vi "Save Waveform To File.vi"(8 "error in":errorcluster, 10 "Waveforms":waveform(dbl)[](array[waveform]), 11 "Measurement Configuration In":T1={"TDMS File Location"="", "Run Action"="Create/Replace Wfm Group", "Wfm Group Name"="Wfm1", "Channel Names"=[], "Waveforms Summary JSON"=[]}) -> (0 "error out":errorcluster, 2 "Final Wfm Group Name":string, 3 "Measurement Configuration Out":T1)   [LabVIEW 2025, in "TDMS Waveform Creator.lvclass"]
uses:
  TDMS Waveform Creator.lvclass
  TDMS Waveform Creator.lvclass/TDMS Waveform Creator.ctl
  <vilib>/regexp/Match Regular Expression.xnode
  <vilib>/ErrorRing/Error Ring.xnode
  <vilib>/Utility/error.llb/Error Cluster From Error Code.vi
  Measurement Configuration.ctl
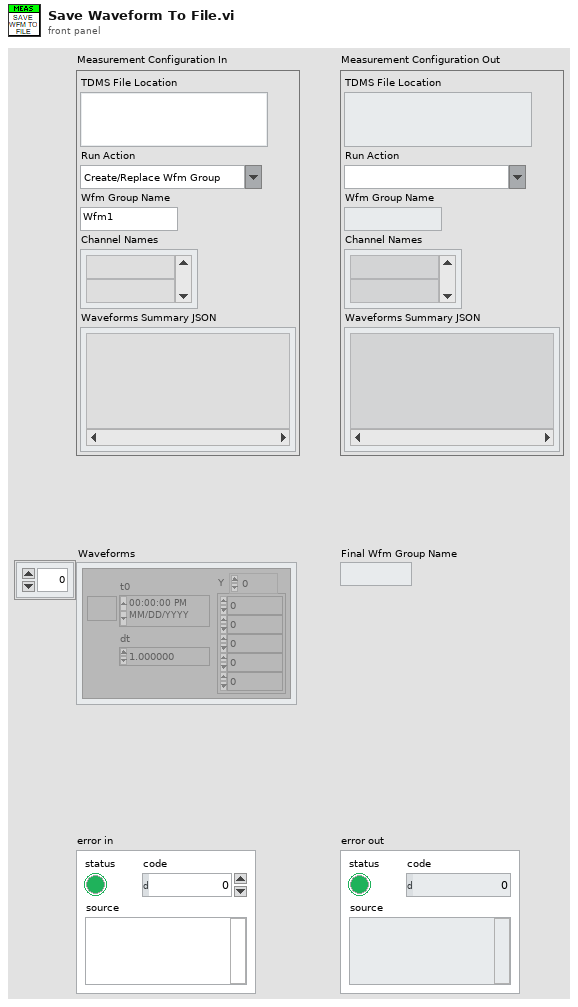
[diagram p1: front panel]
types:
  T1 = typedef "TDMS Waveform Creator.lvclass/Measurement Configuration.ctl" = cluster{"TDMS File Location":string, "Run Action":string, "Wfm Group Name":string, "Channel Names":string[], "Waveforms Summary JSON":string[]}
  T2 = enum16{"open", "open or create", "create or replace", "create", "open (read-only)"}
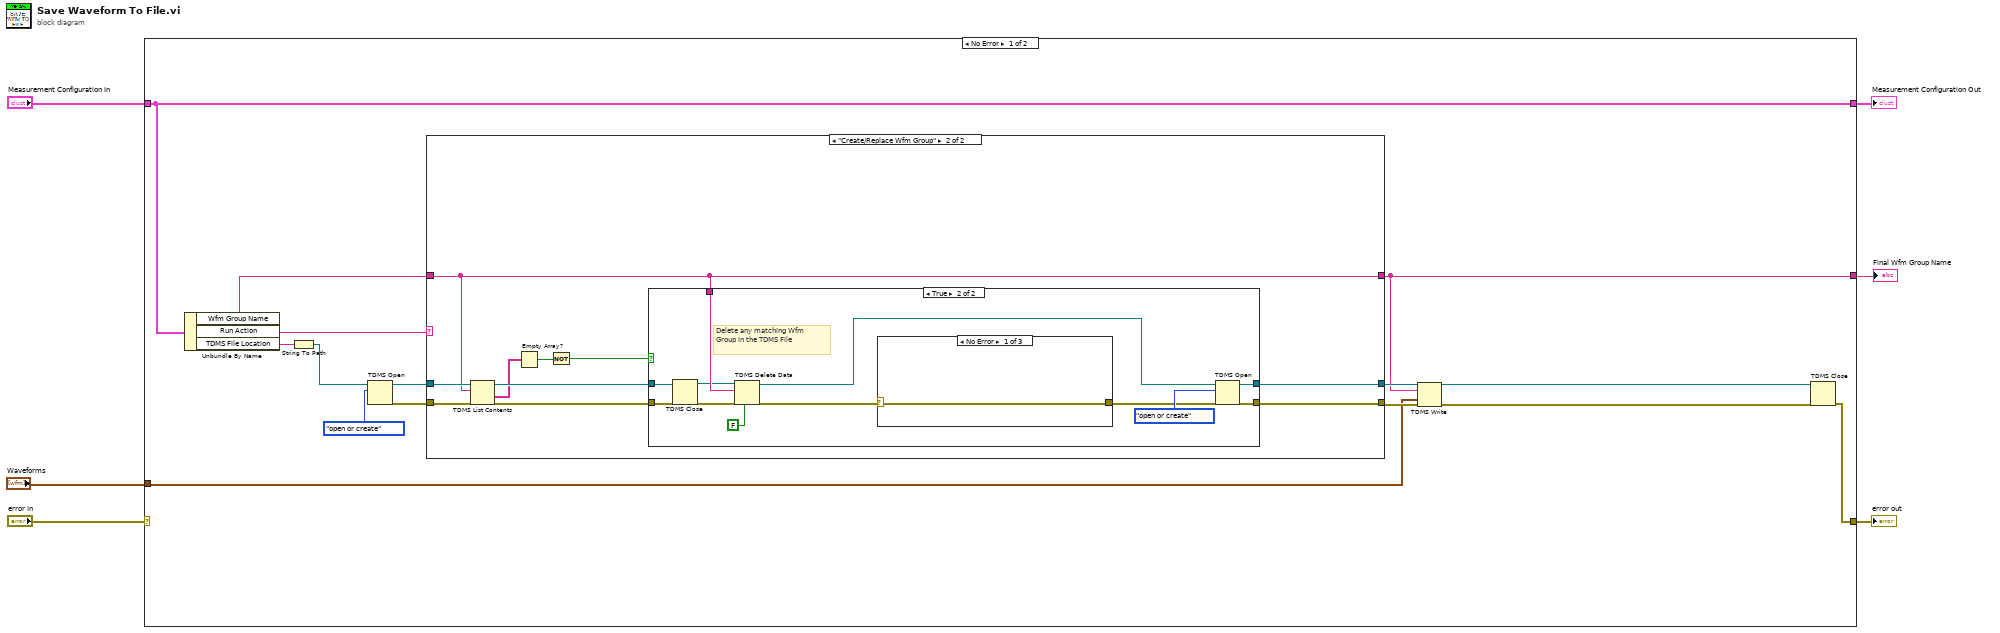
[diagram p0: block diagram]
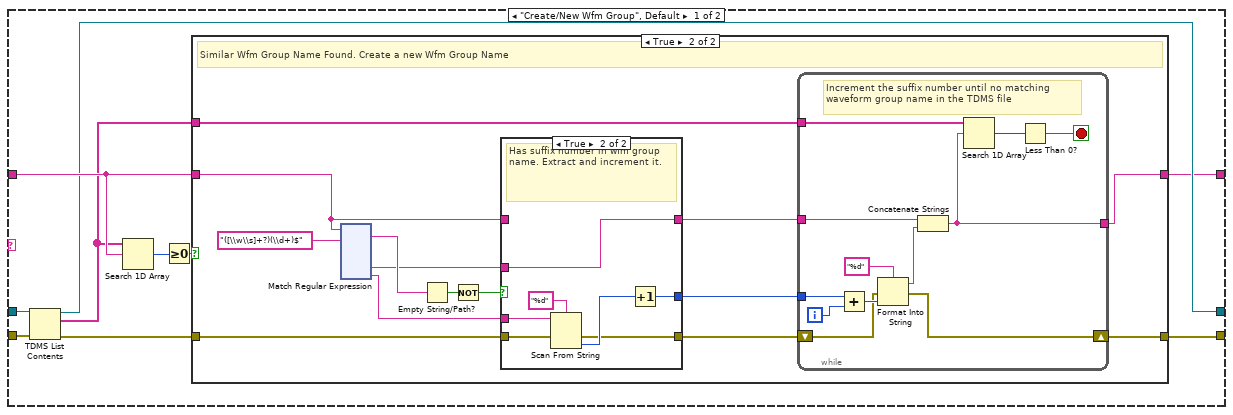
[diagram p2: hidden frame]
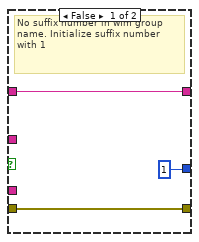
[diagram p4: hidden frame]
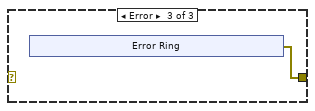
[diagram p7: hidden frame]
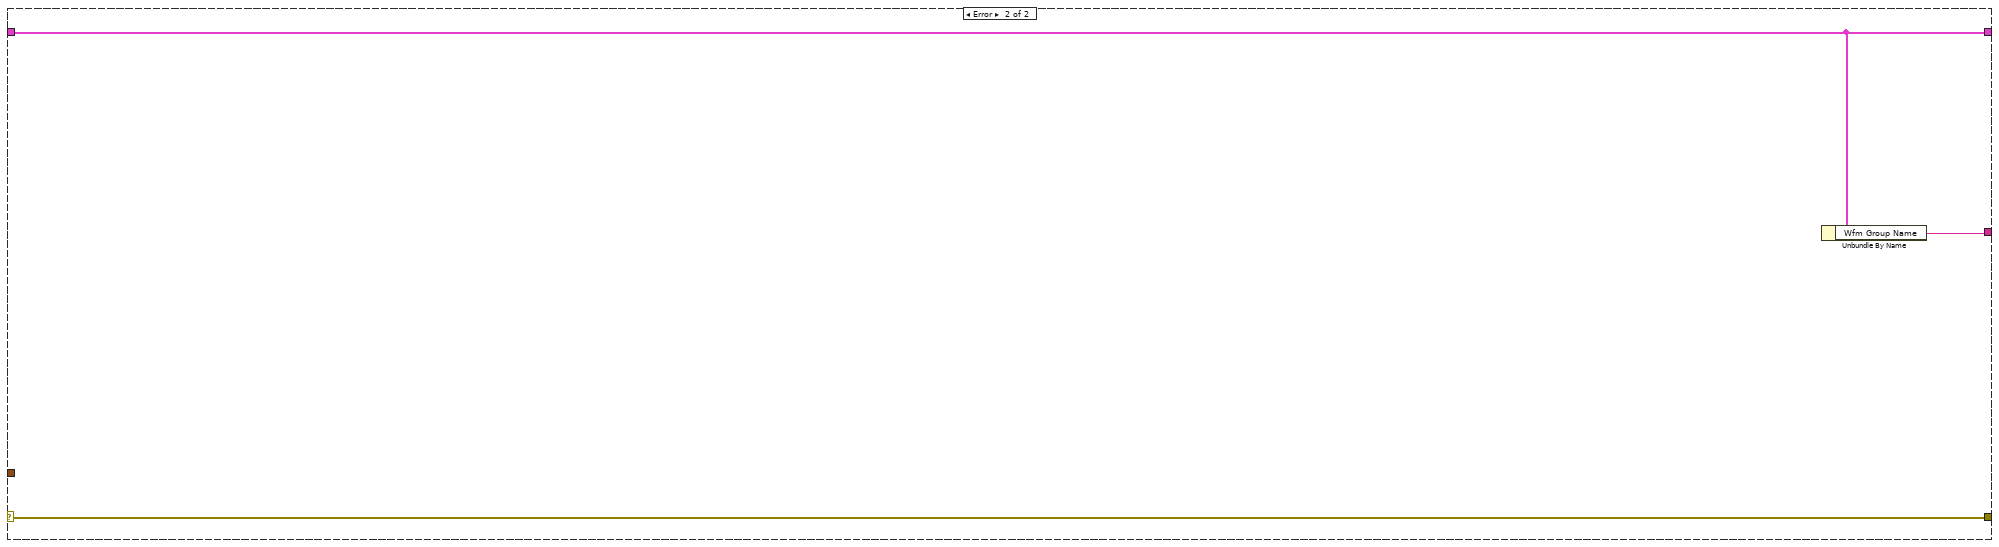
[diagram p8: hidden frame]
diagram:
  n1 = case shown="No Error" "error in" {
    selector: "error in" -> [_ w224]
    tunnel: [w8 w224] -> w5
    tunnel: "Measurement Configuration In" -> [w14 w223]
    tunnel: [w14 w223] -> w3
    tunnel: "Waveforms" -> [w11 _]
    tunnel: [w7 w222] -> w1
    frame No Error {
      n2 = Unbundle By Name(w14) -> ("Wfm Group Name"=w19:string, "Run Action"=w20:string, "TDMS File Location"=w21:string)
      n3 = String To Path(string=w21) -> (path=w18:path)
      n4 = TDMS Open(10:T2."open or create" ("operation (0:open)"), 11:w18) -> (0:w16:errorcluster, 3:w15:refnum<k34>)  [unwired: 5 in]
      n5 = case shown="\"Create/Replace Wfm Group\"" w20 {
        tunnel: w19 -> [w29 w193]
        tunnel: [w26 w198] -> w13
        tunnel: [w25 w199] -> w12
        tunnel: w16 -> [w24 w197]
        tunnel: w15 -> [w23 w195]
        tunnel: [w22 w193] -> w7
        frame "Create/New Wfm Group", Default {
          n6 = TDMS List Contents(4:w24, 7:w23) -> (0:w27:errorcluster, 2:w28:string[], 3:w26:refnum<k34>)  [unwired: 1 in, 1 out]
          n7 = Search 1D Array(1D array=w28, element=w29) -> (index of element=w30:i32)  [unwired: 1 in]
          n8 = Greater Or Equal To 0?(x=w30) -> (x >= 0?=w31:bool)
          n9 = case shown="True" w31 {
            tunnel: w28 -> [_ w40]
            tunnel: w29 -> [w33 w41]
            tunnel: [w33 w37] -> w22
            tunnel: w27 -> [w32 w36]
            tunnel: [w32 w34] -> w25
            frame False {
              # "No clash of Wfm Group Name"
            }
            frame True {
              # "Similar Wfm Group Name Found. Create a new Wfm Group Name"
              n10 = xnode "Match Regular Expression"("input string"=w41, "regular expression"="([\\w\\s]+?)(\\d+)$") -> ("whole match"=w46:string, "submatch 1"=w42:string, "submatch 2"=w45:string)  [unwired: 4 in, 4 out]
              n11 = Empty String/Path?(string/path=w46) -> (empty?=w43:bool)
              n12 = Not(x=w43) -> (.not. x?=w38:bool)
              n13 = case shown="True" w38 {
                tunnel: w45 -> [_ w57]
                tunnel: [1 w54] -> w44
                tunnel: w42 -> [_ w53]
                tunnel: w41 -> [w50 _]
                tunnel: [w50 w53] -> w39
                tunnel: w36 -> [w48 w52]
                tunnel: [w48 w51] -> w35
                frame False {
                  # "No suffix number in wfm group name. Initialize suffix number with 1"
                }
                frame True {
                  # "Has suffix number in wfm group name. Extract and increment it."
                  n14 = Scan From String(format string="%d", input string=w57, error in=w52) -> (error out=w51:errorcluster, output 1=w55:i32)  [unwired: 2 in, 2 out]
                  n15 = Increment(x=w55) -> (x+1=w54:i32)
                }
              }
              n16 = while {
                tunnel: w44 -> [w68]
                tunnel: w40 -> [w67]
                tunnel: [w61] -> w37
                tunnel: w39 -> [w60]
                shift-right: [w58] -> w34
                shift-left: w35 -> [w59]
                i -> [w69]
                stop <- w62 stop-if-true
                # "Increment the suffix number until no matching waveform group name in the TDMS file"
                n17 = Add(x=w68, y=w69) -> (x+y=w66:i32)
                n18 = Format Into String(format string="%d", error in=w59, w66) -> (resulting string=w64:string, error out=w58:errorcluster)  [unwired: 1 in]
                n19 = Concatenate Strings(w60, w64) -> (w61:string)
                n20 = Search 1D Array(1D array=w67, element=w61) -> (index of element=w63:i32)  [unwired: 1 in]
                n21 = Less Than 0?(x=w63) -> (x < 0?=w62:bool)
              }
            }
          }
        }
        frame "Create/Replace Wfm Group" {
          n22 = TDMS List Contents(4:w197, 6:w193, 7:w195) -> (0:w196:errorcluster, 1:w190:string[], 3:w194:refnum<k34>)  [unwired: 1 out]
          n23 = Empty Array?(array=w190) -> (empty?=w192:bool)
          n24 = Not(x=w192) -> (.not. x?=w191:bool)
          n25 = case shown="True" w191 {
            tunnel: [w200 w213] -> w199
            tunnel: [w201 w212] -> w198
            tunnel: w196 -> [w200 w211]
            tunnel: w194 -> [w201 w210]
            tunnel: w193 -> [_ w209]
            frame False {
            }
            frame True {
              # "Delete any matching Wfm Group in the TDMS File"
              n26 = TDMS Close(8:w211, 11:w210) -> (0:w206:errorcluster, 3:w207:path)
              n27 = TDMS Delete Data(6:FALSE ("keep empty group/channel? (T)"), 8:w206, 10:w209, 11:w207) -> (0:w204:errorcluster, 3:w205:path)  [unwired: 3 in]
              n28 = case shown="No Error" w204 {
                selector: w204 -> [w214 w215 _]
                tunnel: [w214 w215 w216] -> w203
                frame No Error {
                }
                frame Default {
                }
                frame Error {
                  n29 = xnode "Error Ring"() -> ("error out"=w216:errorcluster)
                }
              }
              n30 = TDMS Open(8:w203, 10:T2."open or create" ("operation (0:open)"), 11:w205) -> (0:w213:errorcluster, 3:w212:refnum<k34>)  [unwired: 4 in]
            }
          }
        }
      }
      n31 = TDMS Write(0:w13, 5:w7, 9:w11, 11:w12) -> (4:w10:refnum<k34>, 15:w9:errorcluster)  [unwired: 2 in, 2 out]
      n32 = TDMS Close(8:w9, 11:w10) -> (0:w8:errorcluster)  [unwired: 1 out]
    }
    frame Error {
      n33 = Unbundle By Name(w223) -> ("Wfm Group Name"=w222:string)
    }
  }
  "error out" <- w5
  "Measurement Configuration Out" <- w3
  "Final Wfm Group Name" <- w1
